vi "BasicVIDocumentation_Interface.vi"(9 "EventsIn":T1, 10 "Events":T2) -> ()   [LabVIEW 2014, in "BasicVIDocumentation.lvlib" / "BasicVIDocumentation.lvclass"]
uses:
  BasicVIDocumentation.lvclass
  Framework/_Plugins/_LVCMPlugin/GCMPlugin_EventsOut.ctl
  Framework/_Plugins/_LVCMPlugin/GCMPlugin_EventsIn.ctl
  <vilib>/LabVIEW Icon API/LabVIEW Icon API.lvlib
  Framework/_Plugins/GCMPlugin/GCMPlugin.lvclass
panel:
  out "Icon":picture
  in  "Description":string
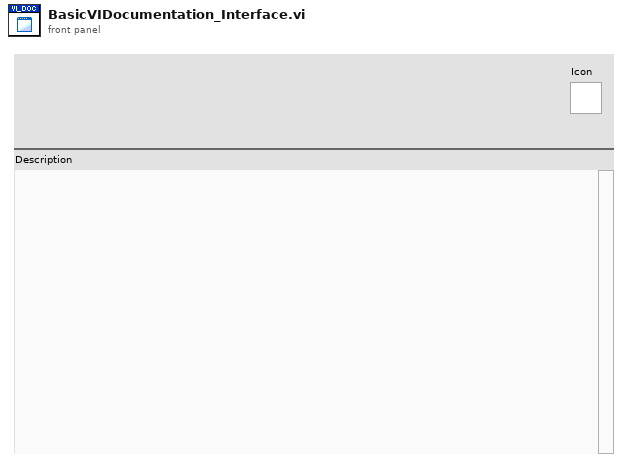
[diagram p1: front panel]
types:
  T1 = typedef "GCMPlugin.lvclass/GCMPlugin_EventsIn.ctl" = cluster{"Stop":refnum<user-event>, "ItemSelected":refnum<user-event>, "ItemDeselected":refnum<user-event>, "PluginActivated":refnum<user-event>, "PluginDeactivated":refnum<user-event>}
  T2 = typedef "GCMPlugin.lvclass/GCMPlugin_EventsOut.ctl" = cluster{"ItemEdited":refnum<user-event>}
  T3 = typedef "imagedata.ctl" = cluster{"image type":i32, "image depth":i32, "image":u8[], "mask":u8[], "colors":u32[], "Rectangle":cluster{"left":i16, "top":i16, "right":i16, "bottom":i16}}
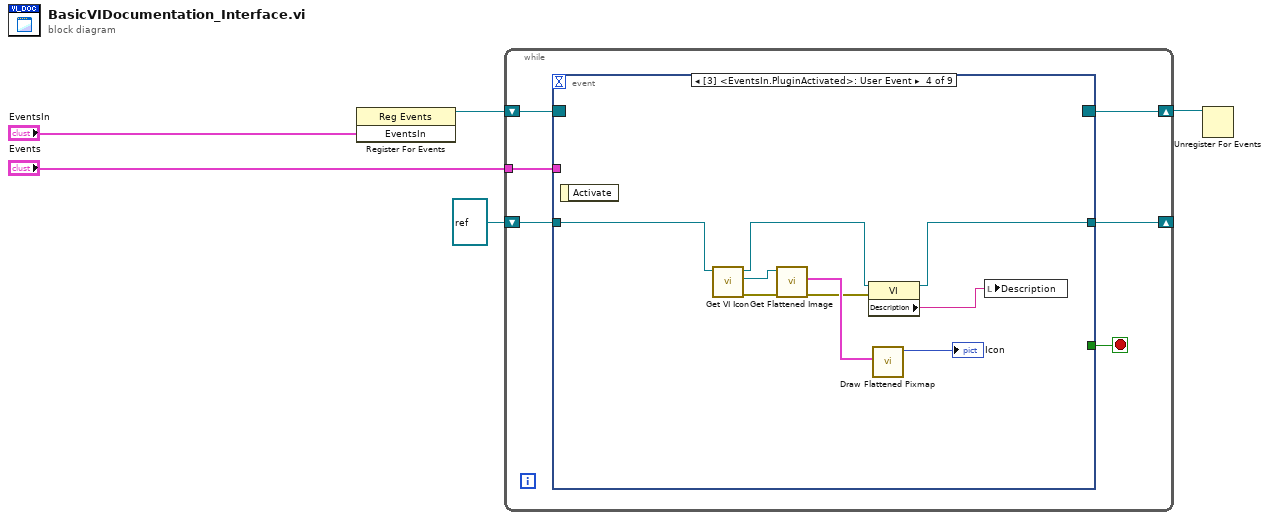
[diagram p0: block diagram]
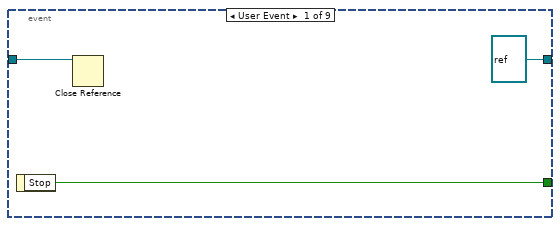
[diagram p2: hidden frame]
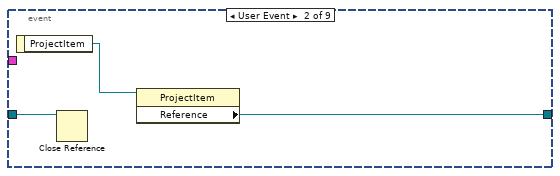
[diagram p3: hidden frame]
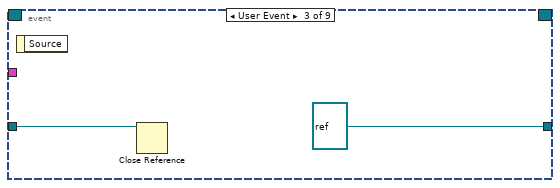
[diagram p4: hidden frame]
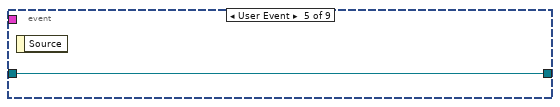
[diagram p5: hidden frame]
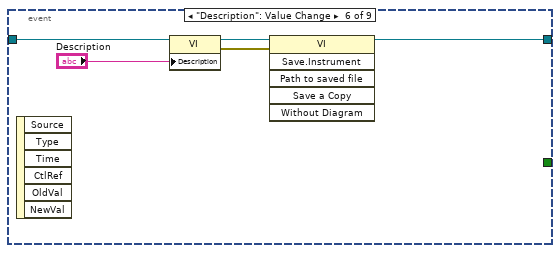
[diagram p6: hidden frame]
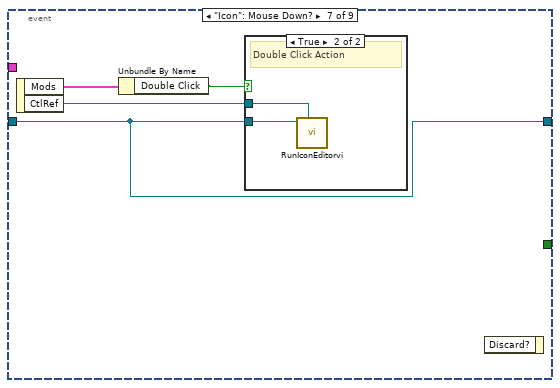
[diagram p7: hidden frame]
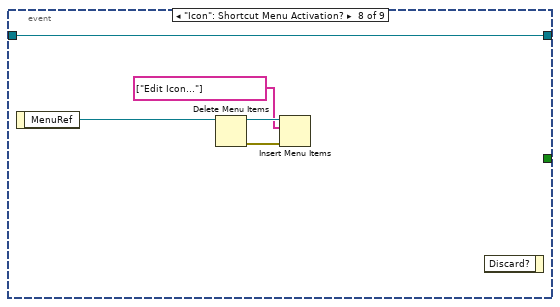
[diagram p9: hidden frame]
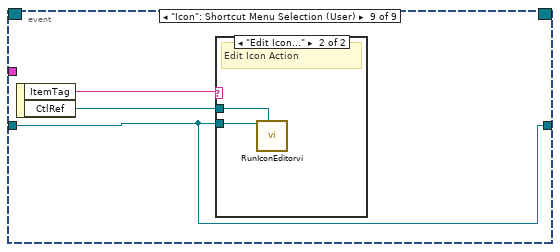
[diagram p10: hidden frame]
diagram:
  n1 = register-events("EventsIn") -> (reference out=w4:refnum<event-registration>)  [unwired: 2 in, 1 out]
  n2 = while {
    tunnel: "Events" -> [w10]
    shift-right: [w7] -> w2
    shift-left: w4 -> [w11]
    shift-right: [w6] -> _
    shift-left: refnum<vi> refnum ("VI Refnum out") -> [w8]
    stop <- w9 stop-if-true
    n3 = event shown="[3] <EventsIn.PluginActivated>: User Event" {
      selector: w11 -> [_ _ _ _ _ _ _ _ _]
      dyn-events: [_ _ _ _ _ _ _ _ _] -> w7
      timeout: _ -> [_ _ _ _ _ _ _ _ _]
      tunnel: w10 -> [_ _ _ _ _ _ _ _ _]
      tunnel: [w14 _ _ _ _ _ _ _ _] -> w9
      tunnel: w8 -> [w13 w16 w19 w24 w29 w34 w35 w41 w46]
      tunnel: [refnum<vi> refnum ("VI Refnum out") w15 refnum<vi> refnum ("VI Refnum out") w21 w29 w31 w35 w41 w46] -> w6
      event User Event {
        n4 = event-data() -> ("Stop"=w14:bool)  [unwired: 1 in]
        n5 = Close Reference(reference=w13) -> ()  [unwired: 1 in, 1 out]
      }
      event User Event {
        n6 = event-data() -> ("ProjectItem"=w17:refnum<vi>)  [unwired: 1 in]
        n7 = Close Reference(reference=w16) -> ()  [unwired: 1 in, 1 out]
        n8 = property class="ProjectItem"(reference=w17) -> ("Reference"=w15:refnum<vi>)  [unwired: 1 in, 2 out]
      }
      event User Event {
        n9 = event-data() -> ()  [unwired: 1 in, 1 out]
        n10 = Close Reference(reference=w19) -> ()  [unwired: 1 in, 1 out]
      }
      event User Event {
        n11 = event-data() -> ()  [unwired: 1 in, 1 out]
        n12 = call <vilib>:"Get VI Icon.vi"("VI Refnum in"=w24) -> ("error out"=w26:errorcluster, "Icon"=w25:refnum<class "Icon.lvclass">, "VI Refnum out"=w22:refnum<vi>)  [unwired: 8 in]
        n13 = call <vilib>:"Get Flattened Image.vi"("error in (no error)"=w26, "lv_icon.lvlib:Icon.lvclass in"=w25) -> ("error out"=w23:errorcluster, "Color Image"=w27:T3)  [unwired: 6 in, 2 out]
        n14 = property class="VI"(reference=w22, error in=w23) -> (reference out=w21:refnum<vi>, "Description"=w20:string)  [unwired: 1 out]
        n15 = call <vilib>:"Draw Flattened Pixmap.vi"("image data"=w27) -> ("new picture"=→"Icon":picture)  [unwired: 8 in]
        n16 = local write "Description"(w20) -> ()
      }
      event User Event {
        n17 = event-data() -> ()  [unwired: 1 in, 1 out]
      }
      event "Description": Value Change {
        n18 = event-data() -> ()  [unwired: 1 in, 6 out]
        n19 = property class="VI"(reference=w34, "Description"="Description") -> (reference out=w33:refnum<vi>, error out=w32:errorcluster)  [unwired: 1 in]
        n20 = invoke class="VI" method="Save.Instrument"(reference=w33, error in=w32) -> (reference out=w31:refnum<vi>)  [unwired: 4 in, 5 out]
      }
      event "Icon": Mouse Down? {
        n21 = event-data() -> ("Mods"=w38:cluster{"Double Click":bool, "Menu Key":bool}, "CtlRef"=w36:refnum<vi>)  [unwired: 1 in]
        n22 = Unbundle By Name(w38) -> ("Double Click"=w37:bool)
        n23 = case shown="True" w37 {
          tunnel: w35 -> [_ w40]
          tunnel: w36 -> [_ w39]
          frame False {
            # "Single Click Action"
          }
          frame True {
            # "Double Click Action"
            n24 = call "RunIconEditorvi.vi"("CtlRef"=w39, "VI Refnum in"=w40) -> ()  [unwired: 9 in, 1 out]
          }
        }
        n25 = event-data() -> ()  [unwired: 2 in, 1 out]
      }
      event "Icon": Shortcut Menu Activation? {
        n26 = event-data() -> ("MenuRef"=w45:refnum<k9>)  [unwired: 1 in]
        n27 = Delete Menu Items(9:w45) -> (0:w43:errorcluster, 3:w44:refnum<k9>)  [unwired: 3 in]
        n28 = Insert Menu Items(6:w43, 8:string[] ["Edit Icon..."] ("item names"), 9:w44) -> ()  [unwired: 3 in, 3 out]
        n29 = event-data() -> ()  [unwired: 2 in, 1 out]
      }
      event "Icon": Shortcut Menu Selection (User) {
        n30 = event-data() -> ("ItemTag"=w48:string, "CtlRef"=w47:refnum<vi>)  [unwired: 1 in]
        n31 = case shown="\"Edit Icon...\"" w48 {
          tunnel: w46 -> [_ w50]
          tunnel: w47 -> [_ w49]
          frame "False", Default {
            # "Default Action"
          }
          frame "Edit Icon..." {
            # "Edit Icon Action"
            n32 = call "RunIconEditorvi.vi"("CtlRef"=w49, "VI Refnum in"=w50) -> ()  [unwired: 9 in, 1 out]
          }
        }
      }
    }
  }
  n33 = Unregister For Events(event registration refnum=w2) -> ()  [unwired: 1 in, 1 out]
